vi "Diagnostics SysDef Example.vi"() -> (0 "error out":errorcluster)   [LabVIEW 2015]
uses:
  Diagnostics SysDef API.lvlibp/addons/Diagnostics/Source/System Explorer/Types/SysDef.Export.ctl
  Diagnostics SysDef API.lvlibp/addons/Diagnostics/Source/Shared/Types/CAN.ctl
  Diagnostics SysDef API.lvlibp/addons/Diagnostics/Source/Shared/Types/CAN.Interface.ctl
  Diagnostics SysDef API.lvlibp/addons/Diagnostics/Source/Shared/Types/Protocol.ctl
  Diagnostics SysDef API.lvlibp/addons/Diagnostics/Source/Shared/Types/Transport.ctl
  Diagnostics SysDef API.lvlibp/addons/Diagnostics/Source/Shared/Types/Security.ctl
  Diagnostics SysDef API.lvlibp/addons/Diagnostics/Source/System Explorer/Types/Frames.Export.ctl
  Diagnostics SysDef API.lvlibp/addons/Diagnostics/Source/System Explorer/Types/Frame.Export.ctl
  Diagnostics SysDef API.lvlibp/addons/Diagnostics/Source/Shared/Types/Signal.ctl
  Diagnostics SysDef API.lvlibp/addons/Diagnostics/Source/System Explorer/Types/DPIDs.Export.ctl
  Diagnostics SysDef API.lvlibp/addons/Diagnostics/Source/System Explorer/Types/DPID.Export.ctl
  Diagnostics SysDef API.lvlibp/addons/Diagnostics/Source/Shared/Types/DPID.ctl
  Diagnostics SysDef API.lvlibp/addons/Diagnostics/Source/Shared/Types/DPID.Rate.ctl
  Diagnostics SysDef API.lvlibp/addons/Diagnostics/Source/System Explorer/Types/DTC.Export.ctl
  Diagnostics SysDef API.lvlibp/addons/Diagnostics/Source/Shared/Types/DTCDescriptor.ctl
  Diagnostics SysDef API.lvlibp/addons/Diagnostics/Source/System Explorer/Types/DTCControl.Export.ctl
  Diagnostics SysDef API.lvlibp/addons/Diagnostics/Source/Shared/Types/986x.ctl
  Diagnostics SysDef API.lvlibp/addons/Diagnostics/Source/System Explorer/Types/Command.Export.ctl
  Diagnostics SysDef API.lvlibp/addons/Diagnostics/Source/System Explorer/Types/Status.Export.ctl
  Diagnostics SysDef API.lvlibp/addons/Diagnostics/Source/System Explorer/Types/IOControls.Export.ctl
  Diagnostics SysDef API.lvlibp/addons/Diagnostics/Source/System Explorer/Types/IO.Export.ctl
  Diagnostics SysDef API.lvlibp/addons/Diagnostics/Source/System Explorer/Types/CmdResp.Export.ctl
  Diagnostics SysDef API.lvlibp/addons/Diagnostics/Source/System Explorer/Types/Routines.Export.ctl
  Diagnostics SysDef API.lvlibp/addons/Diagnostics/Source/System Explorer/Types/Routine.Export.ctl
  Diagnostics SysDef API.lvlibp/addons/Diagnostics/Source/System Explorer/Types/UserDefined.Export.ctl
  Diagnostics SysDef API.lvlibp/addons/Diagnostics/Source/System Explorer/Types/UserDefined.Group.Export.ctl
  Diagnostics SysDef API.lvlibp/addons/Diagnostics/Source/System Explorer/Types/UserDefined.Group.Message.Export.ctl
  NationalInstruments.VeriStand.Internal
  NationalInstruments.VeriStand.SystemDefinitionAPI
  Diagnostics SysDef API.lvlibp
  Diagnostics SysDef API.lvlibp/addons/Diagnostics/Source/Shared/Diagnostics Addon Shared.lvlib
  Diagnostics SysDef API.lvlibp/addons/Diagnostics/Source/System Explorer/Diagnostics Addon System Explorer.lvlib
panel:
  in  "Configuration":T1={"Name"="Diagnostic Addon", "Description"="", "Diagnostics Basic Configuraiton"={"CAN Interface"=enum."CAN0", "Baud Rate"=0, "Diagnostic Protocol"=enum."GMLAN", "Transport Protocol"=enum."ISO TP - Normal Mode", "Transmit ID"=0, "Receive ID"=0, "Transmit Extension"=0, "Receive Extension"=0, "Receive UUDT ID"=0, "Enable Stream"=TRUE, "VW TP Channel ID"=0, "Security"={"Source DLL Path"=path "", "Security Level"=1, "Target DLL Path"=path ""}, "Fill Frame"=FALSE, "Fill Byte"=255, "Termination"=FALSE}, "DID Outputs"={"Description"="", "Frames"=[]}, "DID Inputs"={"Description"="", "Frames"=[]}, "PID Outputs"={"Description"="", "Frames"=[]}, "PID Inputs"={"Description"="", "Frames"=[]}, "DPIDs"={"Description"="", "DPIDs"=[]}, "DTC"={"Description"="", "DTC descriptor"={"DTC Byte Length"=2, "Status Byte Length"=1, "Add Data Byte Length"=1, "Byte Order"=enum."Motorola"}, "DTC Control"={"Description"="", "Signals"=[]}, "Created DTCs"=0}, "NI 986x Support"={"Enable"=FALSE, "RIO Device"=0, "Bitfile"=path ""}, "Commands"={"Description"=""}, "Status"={"Description"=""}, "IO Controls"={"Description"="", "IO Control Array"=[]}, "Routines"={"Description"="", "Routine Array"=[]}, "Memory Outputs"={"Description"="", "Frames"=[]}, "Memory Inputs"={"Description"="", "Frames"=[]}, "User Defined"={"Description"="", "Groups"=[]}} {"DID Outputs"."Frames"."Signals"."Byte Order" items=["Little Endian", "Big Endian"]; "DID Outputs"."Frames"."Signals"."Data Type" items=["Signed", "Unsigned", "IEEE Float"]; "Memory Inputs"."Frames"."Signals"."Byte Order" items=["Little Endian", "Big Endian"]; "Memory Inputs"."Frames"."Signals"."Data Type" items=["Signed", "Unsigned", "IEEE Float"]; "Memory Outputs"."Frames"."Signals"."Byte Order" items=["Little Endian", "Big Endian"]; "Memory Outputs"."Frames"."Signals"."Data Type" items=["Signed", "Unsigned", "IEEE Float"]; "Routines"."Routine Array"."Stop Parameters"."Response"."Byte Order" items=["Little Endian", "Big Endian"]; "Routines"."Routine Array"."Stop Parameters"."Response"."Data Type" items=["Signed", "Unsigned", "IEEE Float"]; "Routines"."Routine Array"."Stop Parameters"."Cmd"."Byte Order" items=["Little Endian", "Big Endian"]; "Routines"."Routine Array"."Stop Parameters"."Cmd"."Data Type" items=["Signed", "Unsigned", "IEEE Float"]; "Routines"."Routine Array"."Request Parameters"."Response"."Byte Order" items=["Little Endian", "Big Endian"]; "Routines"."Routine Array"."Request Parameters"."Response"."Data Type" items=["Signed", "Unsigned", "IEEE Float"]; "Routines"."Routine Array"."Request Parameters"."Cmd"."Byte Order" items=["Little Endian", "Big Endian"]; "Routines"."Routine Array"."Request Parameters"."Cmd"."Data Type" items=["Signed", "Unsigned", "IEEE Float"]; "Routines"."Routine Array"."Start Parameters"."Response"."Byte Order" items=["Little Endian", "Big Endian"]; "Routines"."Routine Array"."Start Parameters"."Response"."Data Type" items=["Signed", "Unsigned", "IEEE Float"]; "Routines"."Routine Array"."Start Parameters"."Cmd"."Byte Order" items=["Little Endian", "Big Endian"]; "Routines"."Routine Array"."Start Parameters"."Cmd"."Data Type" items=["Signed", "Unsigned", "IEEE Float"]; "IO Controls"."IO Control Array"."Signals"."Response"."Byte Order" items=["Little Endian", "Big Endian"]; "IO Controls"."IO Control Array"."Signals"."Response"."Data Type" items=["Signed", "Unsigned", "IEEE Float"]; "IO Controls"."IO Control Array"."Signals"."Cmd"."Byte Order" items=["Little Endian", "Big Endian"]; "IO Controls"."IO Control Array"."Signals"."Cmd"."Data Type" items=["Signed", "Unsigned", "IEEE Float"]; "DTC"."DTC Control"."Signals"."Byte Order" items=["Little Endian", "Big Endian"]; "DTC"."DTC Control"."Signals"."Data Type" items=["Signed", "Unsigned", "IEEE Float"]; "Diagnostics Basic Configuraiton"."Fill Byte" format="%.0x"; "Diagnostics Basic Configuraiton"."VW TP Channel ID" format="%.0x"; "Diagnostics Basic Configuraiton"."Receive UUDT ID" format="%.0x"; "Diagnostics Basic Configuraiton"."Receive Extension" format="%.0x"; "Diagnostics Basic Configuraiton"."Transmit Extension" format="%.0x"; "Diagnostics Basic Configuraiton"."Receive ID" format="%.0x"; "Diagnostics Basic Configuraiton"."Transmit ID" format="%.0x"; "DID Inputs"."Frames"."Signals"."Byte Order" items=["Little Endian", "Big Endian"]; "DID Inputs"."Frames"."Signals"."Data Type" items=["Signed", "Unsigned", "IEEE Float"]; "PID Inputs"."Frames"."Signals"."Byte Order" items=["Little Endian", "Big Endian"]; "PID Inputs"."Frames"."Signals"."Data Type" items=["Signed", "Unsigned", "IEEE Float"]; "PID Outputs"."Frames"."Signals"."Byte Order" items=["Little Endian", "Big Endian"]; "PID Outputs"."Frames"."Signals"."Data Type" items=["Signed", "Unsigned", "IEEE Float"]}
  in  "error in (no error)":errorcluster
  out "Sysdef Path":path=path "C:/Users/Public/Documents/National Instruments/NI VeriStand 2013/DynamicallyCreatedProject/DynamicallyCreatedProject.nivssdf"
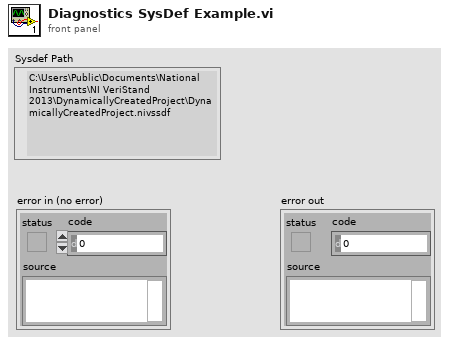
[diagram p1: front panel]
types:
  T1 = typedef "Diagnostics SysDef API.lvlibp/Diagnostics Addon System Explorer.lvlib/SysDef.Export.ctl" = cluster{"Name":string, "Description":string, "Diagnostics Basic Configuraiton":T2, "DID Outputs":T7, "DID Inputs":T7, "PID Outputs":T7, "PID Inputs":T7, "DPIDs":T10, "DTC":T14, "NI 986x Support":T17, "Commands":T18, "Status":T19, "IO Controls":T20, "Routines":T23, "Memory Outputs":T7, "Memory Inputs":T7, "User Defined":T25}
  T2 = typedef "Diagnostics SysDef API.lvlibp/Diagnostics Addon Shared.lvlib/CAN.ctl" = cluster{"CAN Interface":T3, "Baud Rate":u32, "Diagnostic Protocol":T4, "Transport Protocol":T5, "Transmit ID":u32, "Receive ID":u32, "Transmit Extension":u8, "Receive Extension":u8, "Receive UUDT ID":u32, "Enable Stream":bool, "VW TP Channel ID":u32, "Security":T6, "Fill Frame":bool, "Fill Byte":u8, "Termination":bool}
  T3 = typedef "Diagnostics SysDef API.lvlibp/Diagnostics Addon Shared.lvlib/CAN.Interface.ctl" = enum16{"CAN0", "CAN1", "CAN2", "CAN3", "CAN4", "CAN5", "CAN6", "CAN7", "CAN8", "CAN9", "CAN10", "CAN11", "CAN12", "CAN13", "CAN14", "CAN15", "CAN16", "CAN17", "CAN18", "CAN19", "CAN20", "CAN21", "CAN22", "CAN23", "CAN24", "CAN25", "CAN26", "CAN27", "CAN28", "CAN29", "CAN30", "CAN31", "CAN32", "CAN33", "CAN34", "CAN35", "CAN36", "CAN37", "CAN38", "CAN39", "CAN40", "CAN41", "CAN42", "CAN43", "CAN44", "CAN45", "CAN46", "CAN47", "CAN48", "CAN49", "CAN50", "CAN51", "CAN52", "CAN53", "CAN54", "CAN55", "CAN56", "CAN57", "CAN58", "CAN59", "CAN60", "CAN61", "CAN62", "CAN63", "CAN 256 (Virtual)", "CAN 257 (Virtual)"}
  T4 = typedef "Diagnostics SysDef API.lvlibp/Diagnostics Addon Shared.lvlib/Protocol.ctl" = enum16{"GMLAN", "KWP-2000", "UDS", "User-Defined"}
  T5 = typedef "Diagnostics SysDef API.lvlibp/Diagnostics Addon Shared.lvlib/Transport.ctl" = enum16{"ISO TP - Normal Mode", "ISO TP - Mixed Mode", "VW TP 2.0", "Diagnostics on IP"}
  T6 = typedef "Diagnostics SysDef API.lvlibp/Diagnostics Addon Shared.lvlib/Security.ctl" = cluster{"Source DLL Path":path, "Security Level":u8, "Target DLL Path":path}
  T7 = typedef "Diagnostics SysDef API.lvlibp/Diagnostics Addon System Explorer.lvlib/Frames.Export.ctl" = cluster{"Description":string, "Frames":T8[]}
  T8 = typedef "Diagnostics SysDef API.lvlibp/Diagnostics Addon System Explorer.lvlib/Frame.Export.ctl" = cluster{"Name":string, "Description":string, "ID":u32, "Signals":T9[]}
  T9 = typedef "Diagnostics SysDef API.lvlibp/Diagnostics Addon Shared.lvlib/Signal.ctl" = cluster{"Start Bit":u32, "Length":u32, "Scaling Factor":dbl, "Scaling Offset":dbl, "Minimum":dbl, "Maximum":dbl, "Data Type":u32, "Byte Order":u32, "Default Value":dbl, "Name":string, "Units":string, "Description":string}
  T10 = typedef "Diagnostics SysDef API.lvlibp/Diagnostics Addon System Explorer.lvlib/DPIDs.Export.ctl" = cluster{"Description":string, "DPIDs":T11[]}
  T11 = typedef "Diagnostics SysDef API.lvlibp/Diagnostics Addon System Explorer.lvlib/DPID.Export.ctl" = cluster{"Name":string, "Description":string, "DPID":T12}
  T12 = typedef "Diagnostics SysDef API.lvlibp/Diagnostics Addon Shared.lvlib/DPID.ctl" = cluster{"DPID ID":u8, "Speed":T13, "PIDs":u16[]}
  T13 = typedef "Diagnostics SysDef API.lvlibp/Diagnostics Addon Shared.lvlib/DPID.Rate.ctl" = enum16{"Slow", "Medium", "Fast"}
  T14 = typedef "Diagnostics SysDef API.lvlibp/Diagnostics Addon System Explorer.lvlib/DTC.Export.ctl" = cluster{"Description":string, "DTC descriptor":T15, "DTC Control":T16, "Created DTCs":u32}
  T15 = typedef "Diagnostics SysDef API.lvlibp/Diagnostics Addon Shared.lvlib/DTCDescriptor.ctl" = cluster{"DTC Byte Length":i32, "Status Byte Length":i32, "Add Data Byte Length":i32, "Byte Order":enum16{"Motorola", "Intel"}}
  T16 = typedef "Diagnostics SysDef API.lvlibp/Diagnostics Addon System Explorer.lvlib/DTCControl.Export.ctl" = cluster{"Description":string, "Signals":T9[]}
  T17 = typedef "Diagnostics SysDef API.lvlibp/Diagnostics Addon Shared.lvlib/986x.ctl" = cluster{"Enable":bool, "RIO Device":u16, "Bitfile":path}
  T18 = typedef "Diagnostics SysDef API.lvlibp/Diagnostics Addon System Explorer.lvlib/Command.Export.ctl" = cluster{"Description":string}
  T19 = typedef "Diagnostics SysDef API.lvlibp/Diagnostics Addon System Explorer.lvlib/Status.Export.ctl" = cluster{"Description":string}
  T20 = typedef "Diagnostics SysDef API.lvlibp/Diagnostics Addon System Explorer.lvlib/IOControls.Export.ctl" = cluster{"Description":string, "IO Control Array":T21[]}
  T21 = typedef "Diagnostics SysDef API.lvlibp/Diagnostics Addon System Explorer.lvlib/IO.Export.ctl" = cluster{"Name":string, "Description":string, "ID":u16, "Signals":T22}
  T22 = typedef "Diagnostics SysDef API.lvlibp/Diagnostics Addon System Explorer.lvlib/CmdResp.Export.ctl" = cluster{"Cmd":T9[], "Response":T9[]}
  T23 = typedef "Diagnostics SysDef API.lvlibp/Diagnostics Addon System Explorer.lvlib/Routines.Export.ctl" = cluster{"Description":string, "Routine Array":T24[]}
  T24 = typedef "Diagnostics SysDef API.lvlibp/Diagnostics Addon System Explorer.lvlib/Routine.Export.ctl" = cluster{"Name":string, "Description":string, "ID":u16, "Start Parameters":T22, "Request Parameters":T22, "Stop Parameters":T22}
  T25 = typedef "Diagnostics SysDef API.lvlibp/Diagnostics Addon System Explorer.lvlib/UserDefined.Export.ctl" = cluster{"Description":string, "Groups":T26[]}
  T26 = typedef "Diagnostics SysDef API.lvlibp/Diagnostics Addon System Explorer.lvlib/UserDefined.Group.Export.ctl" = cluster{"Name":string, "Description":string, "Messages":T27[]}
  T27 = typedef "Diagnostics SysDef API.lvlibp/Diagnostics Addon System Explorer.lvlib/UserDefined.Group.Message.Export.ctl" = cluster{"Name":string, "Description":string, "Signals":T22}
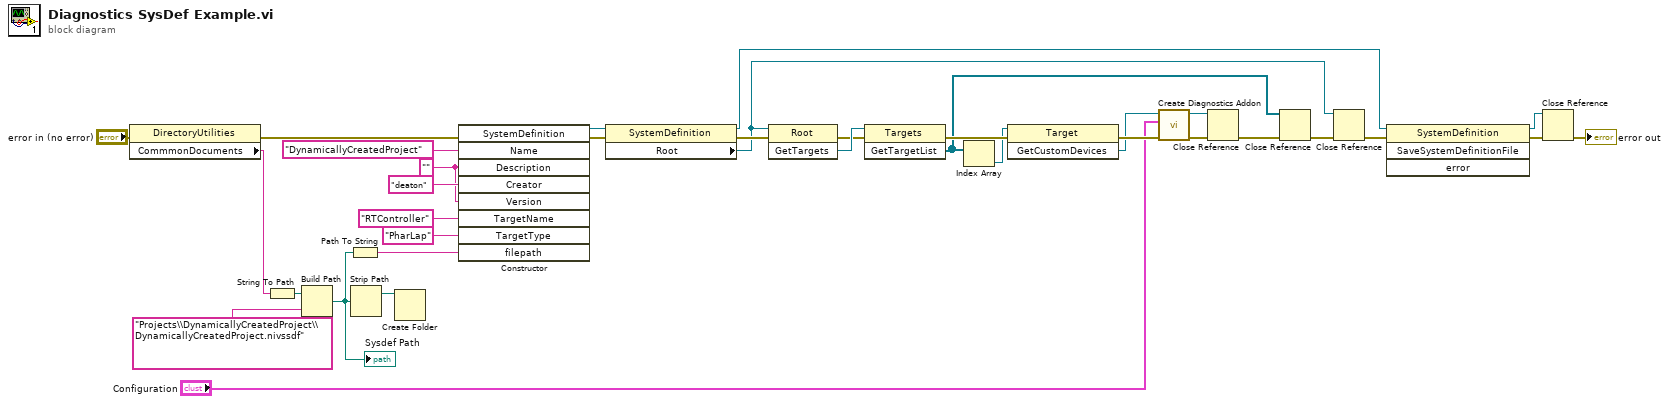
[diagram p0: block diagram]
diagram:
  w31 = "" ("Description")
  n1 = property class="DirectoryUtilities"(error in="error in (no error)") -> (error out=w5:errorcluster, "CommmonDocuments"=w10:string)  [unwired: 1 in, 1 out]
  n2 = String To Path(string=w10) -> (path=w9:path)
  n3 = Build Path(base path=w9, name or relative path="Projects\\DynamicallyCreatedProject\\DynamicallyCreatedProject.nivssdf") -> (appended path=w7:path)
  "Sysdef Path" <- w7
  n4 = Path To String(path=w7) -> (string=w30:string)
  n5 = Strip Path(path=w7) -> (stripped path=w11:path)  [unwired: 1 out]
  n6 = Create Folder(path (use dialog)=w11) -> ()  [unwired: 2 in, 3 out]
  n7 = constructor class="SystemDefinition"(error in=w5, "Name"="DynamicallyCreatedProject", "Description"=w31, "Creator"="deaton", "Version"=w31, "TargetName"="RTController", "TargetType"="PharLap", "filepath"=w30) -> (reference out=w26:refnum<k24>, error out=w28:errorcluster)  [unwired: 2 in, 8 out]
  n8 = property class="SystemDefinition"(reference=w26, error in=w28) -> (reference out=w14:refnum<k24>, error out=w27:errorcluster, "Root"=w13:refnum<k24>)
  n9 = invoke class="Root" method="GetTargets"(reference=w13, error in=w27) -> (error out=w25:errorcluster, "GetTargets"=w29:refnum<k24>)  [unwired: 1 in, 1 out]
  n10 = invoke class="Targets" method="GetTargetList"(reference=w29, error in=w25) -> (error out=w23:errorcluster, "GetTargetList"=w12:refnum<k24>[])  [unwired: 1 in, 1 out]
  n11 = Index Array(array=w12) -> (element=w22:refnum<k24>)  [unwired: 1 in]
  n12 = invoke class="Target" method="GetCustomDevices"(reference=w22, error in=w23) -> (error out=w16:errorcluster, "GetCustomDevices"=w2:refnum<k24>)  [unwired: 1 in, 1 out]
  n13 = call "Create Diagnostics Addon.vi"("error in (no error)"=w16, "Configuration"="Configuration", "Custom Devices Ref"=w2) -> ("error out"=w4:errorcluster, "Custom Devices Ref"=w15:refnum<k24>)  [unwired: 7 in]
  n14 = Close Reference(reference=w15, error in (no error)=w4) -> (error out=w3:errorcluster)
  n15 = Close Reference(reference=w12, error in (no error)=w3) -> (error out=w20:errorcluster)
  n16 = Close Reference(reference=w13, error in (no error)=w20) -> (error out=w21:errorcluster)
  n17 = invoke class="SystemDefinition" method="SaveSystemDefinitionFile"(reference=w14, error in=w21) -> (reference out=w19:refnum<k24>, error out=w17:errorcluster)  [unwired: 2 in, 2 out]
  n18 = Close Reference(reference=w19, error in (no error)=w17) -> (error out=→"error out":errorcluster)
